vi "Feet Per Sec to Deciticks Per Sec.vi"(10 "Ft/Sec":dbl) -> (2 "DeciTick/Sec":dbl)   [LabVIEW 2019]
panel:
  in  "Conversion Factor":dbl=220.0
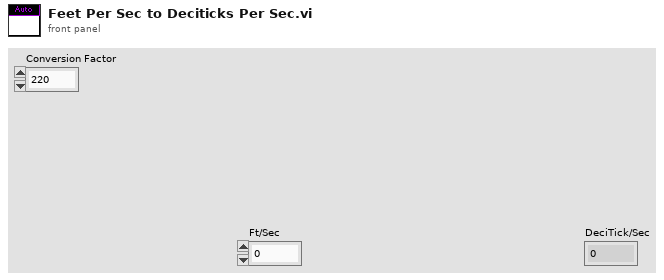
[diagram p1: front panel]
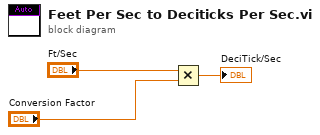
[diagram p0: block diagram]
diagram:
  n1 = Multiply(x="Ft/Sec", y="Conversion Factor") -> (x*y=→"DeciTick/Sec":dbl)
